vi "Dashboard Main.vi"() -> ()   [LabVIEW 2012]
uses:
  <vilib>/event_ctls.llb/eventvkey.ctl
  <vilib>/Utility/config.llb/Read Key (String).vi
  <vilib>/Utility/config.llb/Read Key (I32).vi
  <vilib>/Utility/config.llb/Write Key (String).vi
  <vilib>/Utility/config.llb/Write Key (I32).vi
  <vilib>/Utility/config.llb/NI_LVConfig.lvlib
panel:
  out "Battery Value":dbl(slide) scale=0.0..14.0 scale format="%#_2e"
  out "Battery":sgl(graph)
  in  "Camera Settings":T1={"Frate Rate"=30, "Compression"=30, "Size"=1} {"Frate Rate" scale=1.0..30.0; "Size" items=["640x480", "320x240", "160x120"]}
  out "Mode":T2(ring)=enum."Auto Disabled"
  out "Camera IP":string
  out "JS1 Z":dbl(slide) scale=-1.0..1.0 scale format="%#_2e"
  out "JS2 Z":dbl(slide) scale=-1.0..1.0 scale format="%#_2e"
  out "Alex Left":cluster{"X":dbl, "Y":dbl}[](graph)
  out "Alex Right":cluster{"X":dbl, "Y":dbl}[](graph)
  out "JS Buttons 1":T3
  out "JS Buttons 2":T3
  out "MotorSlide4":dbl(slide) scale=-1.0..1.0 scale format="%#_2e"
  out "MotorSlide3":dbl(slide) scale=-1.0..1.0 scale format="%#_2e"
  out "MotorSlide2":dbl(slide) scale=-1.0..1.0 scale format="%#_2e"
  in  "MotorName3":string="Front Left"
  in  "MotorName4":string="Front Right"
  in  "MotorName1":string="Rear Left"
  in  "MotorName2":string="Rear Right"
  out "MotorChart4":dbl(graph)
  out "MotorChart3":dbl(graph)
  out "MotorChart2":dbl(graph)
  out "MotorSlide1":dbl(slide) scale=-1.0..1.0 scale format="%#_2e"
  out "MotorChart1":dbl(graph)
  out "Robot IP":string
  in  "Dashboard Tab":enum32{"Operation", "Test", "Checklist"}(tab)
  out "Actual RPM":dbl(knob) max=0.0 scale=-500.0..500.0
  out "At Speed?":bool
  in  "Slider":dbl(slide) scale=0.0..100.0 scale format="%#_3g"
  in  "On/Off":bool caption="Solenoid"
  in  "Test Name":u16(ring) items=["Select the test to run...", "Example Test", "-------------------------------", "List of tests is built in robot code.", "Replace with your own automated tests."]
  in  "Test Tree":string(tree)
  in  "Motor":cluster{"Value":dbl, "Enable":bool} {"Value" scale=-1.0..1.0 scale format="%#_3g"}
  out "Progress":T4 {"Test Progress" scale=0.0..100.0}
  in  "Rev/Fwd":cluster{"Forward":bool, "Reverse":bool}
  in  "Ring":u16(ring) items=["Auto", "Fixed indoor", "Fixed outdoor 1", "Fixed outdoor 2", "Fixed fluorescent 1", "Fixed fluorescent 2", "Hold current"]
  in  "Listbox":i32(listbox)
  in  "Viewer":T5(tab)
  out "Mbps":dbl format="%#.1g"
  in  "Enable":bool
  in  "DB Camera Config":bool
  out "Mbps":bool
  out "fps":dbl format="%#.1g"
  out "Image Error Message":string="Timeout in Camera Communications"
  out "Camera Image":T6(plugin-control)
  out "Buttons 1":cluster{"1":bool, "2":bool, "3":bool}
  out "Kinect 1":cluster{"X":dbl, "Y":dbl, "Z":dbl} {"X" scale=1.0..-1.0; "Y" scale=1.0..-1.0; "Z" scale=1.0..-1.0}
  out "Buttons 2":cluster{"1":bool, "2":bool, "3":bool}
  out "Kinect 2":cluster{"X":dbl, "Y":dbl, "Z":dbl} {"X" scale=1.0..-1.0; "Y" scale=1.0..-1.0; "Z" scale=1.0..-1.0}
  out "Version":string
  out "Skeleton Picture":picture
  out "Players":i8
  out "Tree":string(tree)
  # "Drive & Motors"
  # "Robot IP:"
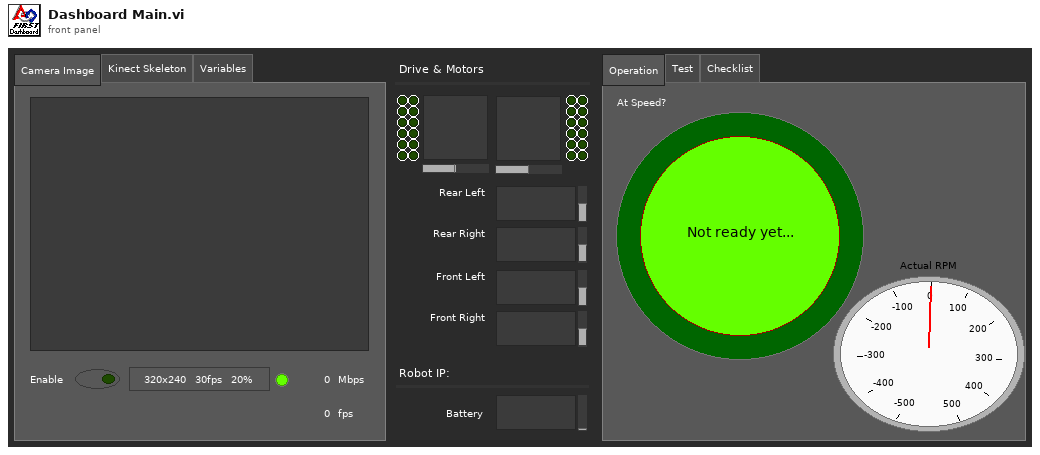
[diagram p1: front panel]
types:
  T1 = cluster{"Frate Rate":i32, "Compression":i32, "Size":u16}
  T2 = enum8{"Tele-Op Disabled", "Tele-Op Enabled", "Auto Disabled", "Auto Enabled", "Test Disabled", "Test Enabled", ""}
  T3 = cluster{bool, bool, bool, bool, bool, bool, bool, bool, bool, bool, bool, bool}
  T4 = cluster{"Test Progress":u8, "Test Progress Text":string}
  T5 = enum32{"Camera Image", "Kinect Skeleton", "Variables"}
  T6 = typedef "IMAQ Image.ctl" = refnum<image>
  T7 = typedef "Image Type" = u32
  T8 = typedef "LVBoundsTypeDef.ctl" = cluster{"Width":u32, "Height":u32}
  T9 = typedef "SkeletonTrackState.ctl" = enum32{"NotTracked", "PositionOnly", "Tracked"}
  T10 = cluster{"TrackingState":u8[], "Position":cluster{"x":sgl, "y":sgl, "z":sgl}, cluster{"x":sgl, "y":sgl, "z":sgl, sgl}[], "TrackState":T9}
  T11 = cluster{cluster{"ScaledToPercentRange":dbl, "ScaledToPercentRange":dbl, "ScaledToPercentRange":dbl}, cluster{bool, bool, bool}}[]
  T12 = cluster{cluster{"ScaledToPercentRange":dbl, "ScaledToPercentRange":dbl, "ScaledToPercentRange":dbl}, cluster{bool, bool, bool}}
  T13 = cluster{"ScaledToPercentRange":dbl, "ScaledToPercentRange":dbl, "ScaledToPercentRange":dbl}
  T14 = typedef "LVRectTypeDef.ctl" = cluster{"Left":i16, "Top":i16, "Right":i16, "Bottom":i16}
  T15 = typedef "NI_LVConfig.lvlib/Config Data RefNum.ctl" = refnum<k1>
  T16 = cluster{"Competition mode":bool, "Robot Link":bool, "Autonomous":bool, "Enabled":bool, "E-Stop":bool, "Simulated":bool, "TestMode":bool, "Docked Window":bool}
  T17 = cluster{"Boolean Array[0]":bool, "Boolean Array[1]":bool, "Boolean Array[2]":bool, "Boolean Array[3]":bool, "Boolean Array[4]":bool, "Boolean Array[5]":bool, "Boolean Array[6]":bool, "Boolean Array[7]":bool, "Boolean Array[8]":bool, "Boolean Array[9]":bool, "Boolean Array[10]":bool, "Boolean Array[11]":bool}
  T18 = typedef "eventvkey.ctl" = enum16{"ASCII", "Enter", "Return", "Shift", "Ctrl", "Alt", "Cmd", "Opt", "Caps", "NumLock", "Clear", "Break", "Up", "Down", "Left", "Right", "Insert", "Delete", "Home", "End", "PageUp", "PageDown", "Escape", "Help", "Pause", "ScrollLock", "F1", "F2", "F3", "F4", "F5", "F6", "F7", "F8", "F9", "F10", "F11", "F12", "F13", "F14", "F15", "F16", "F17", "F18", "F19", "F20", "F21", "F22", "F23", "F24", "Play", "VolumeUp", "VolumeDown", "Mute", "Two Byte Char"}
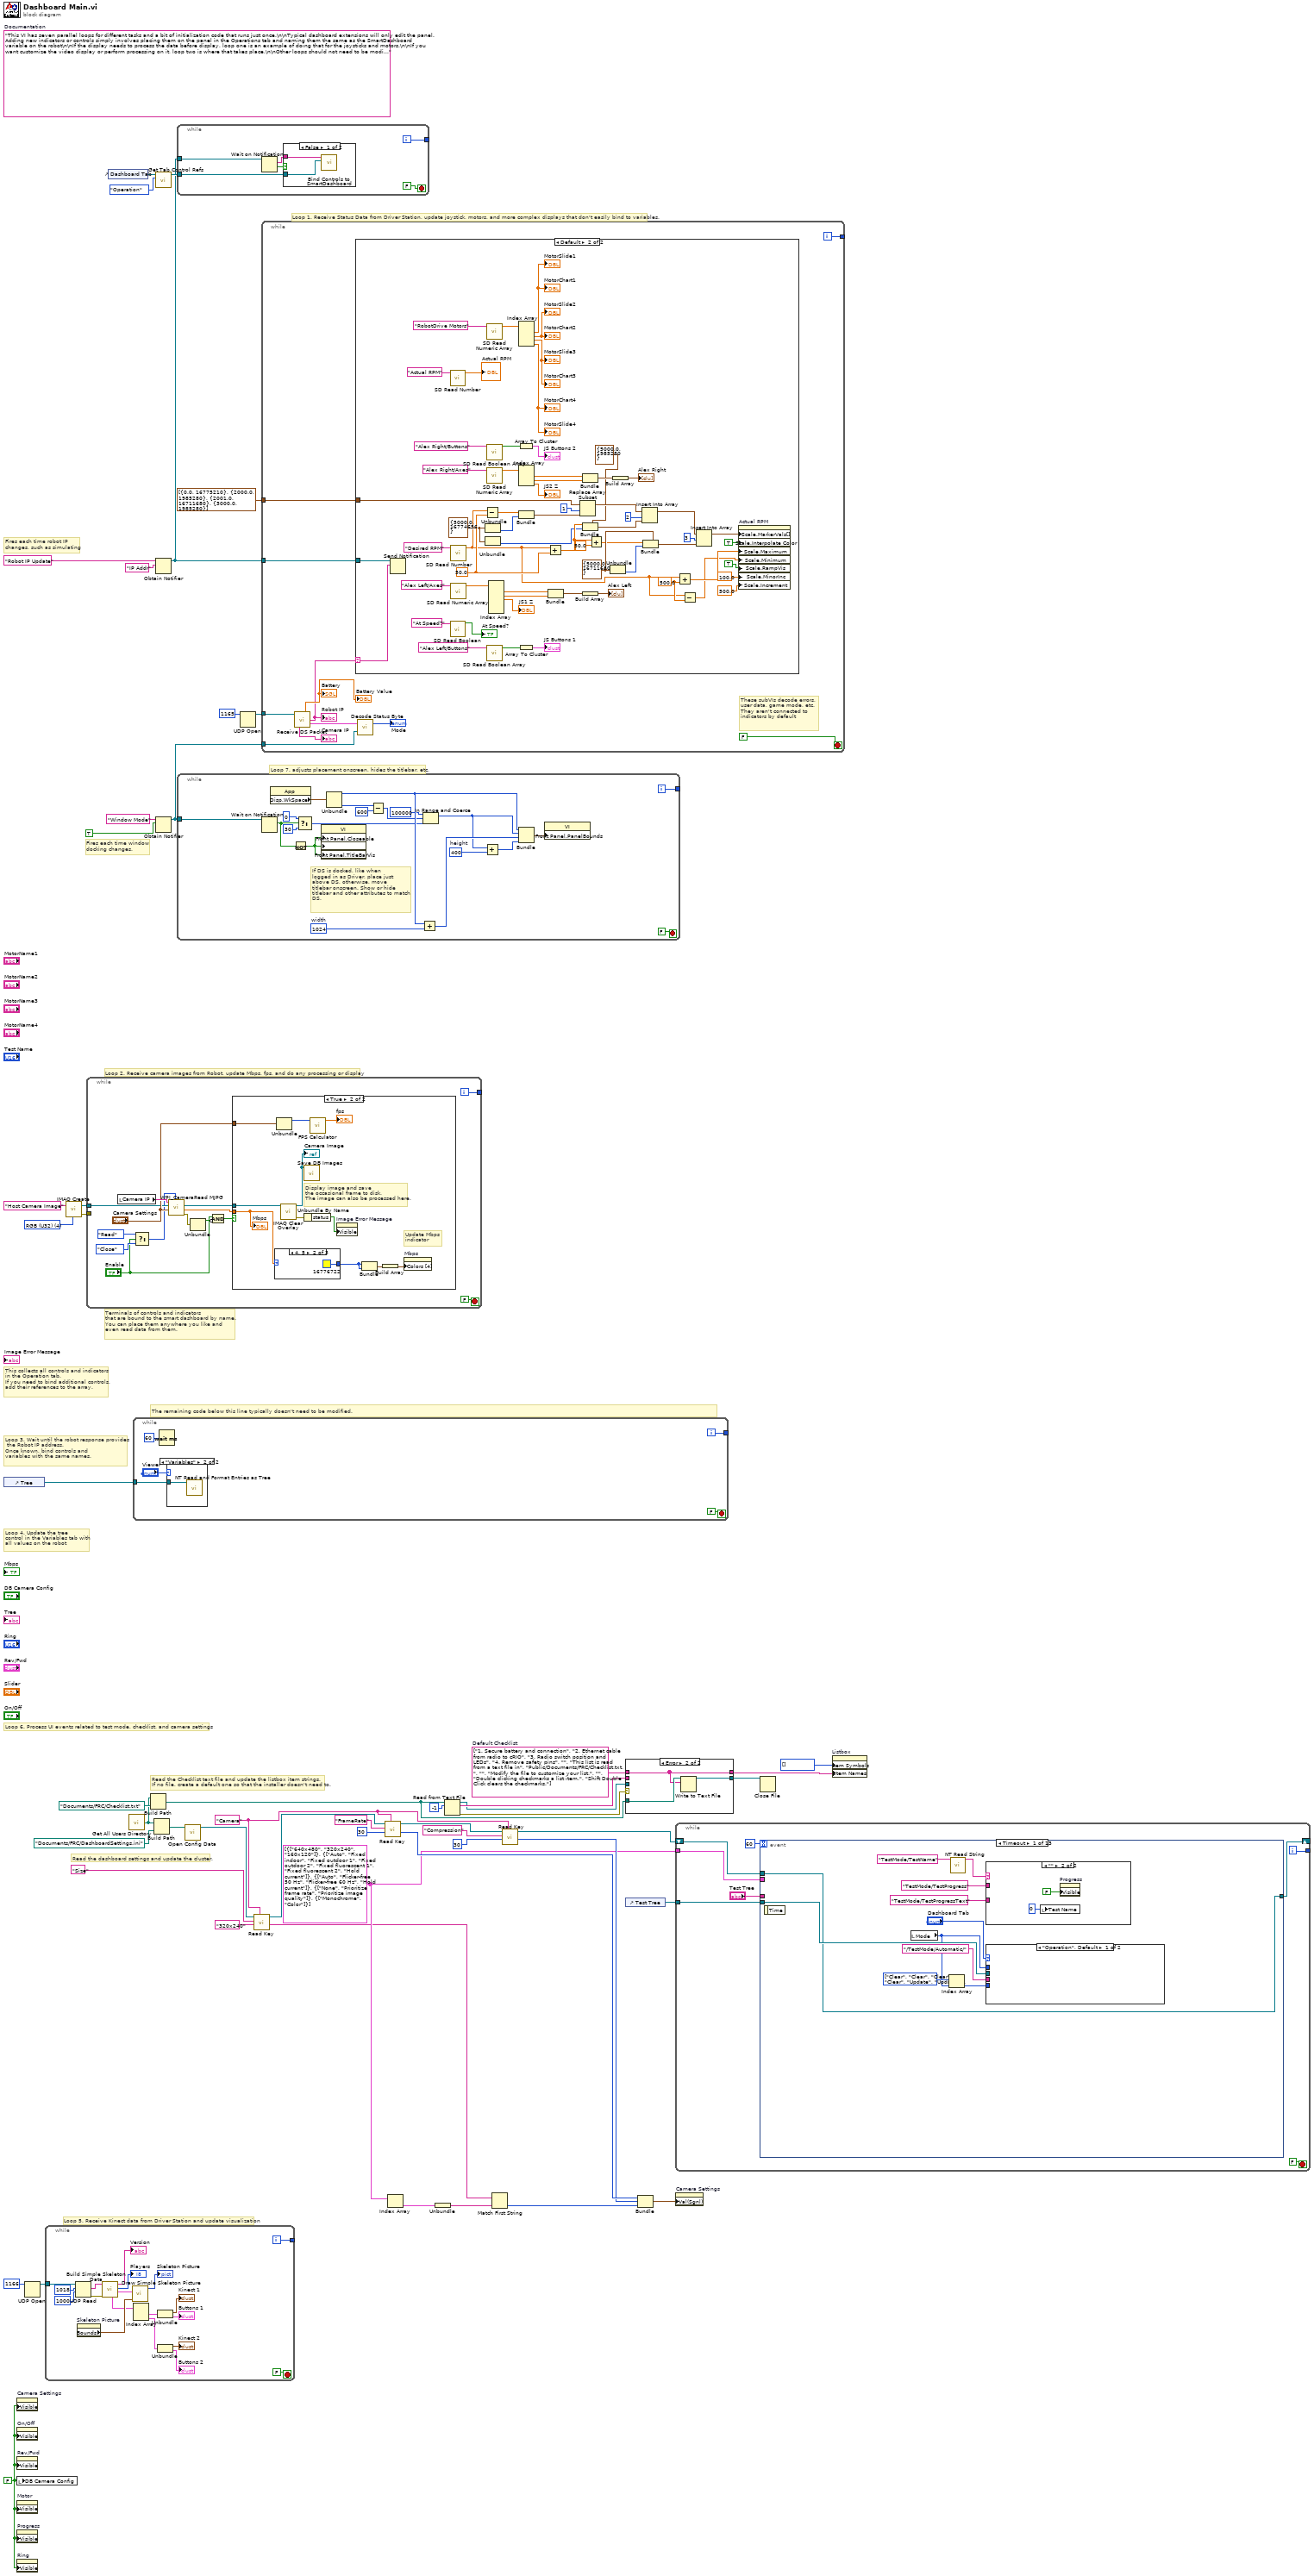
[diagram p0: block diagram]
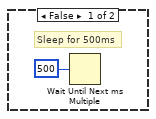
[diagram p3: hidden frame]
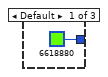
[diagram p4: hidden frame]
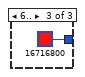
[diagram p5: hidden frame]
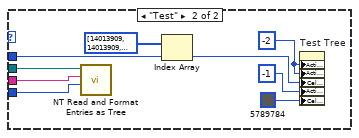
[diagram p7: hidden frame]
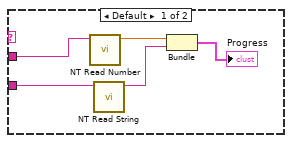
[diagram p8: hidden frame]
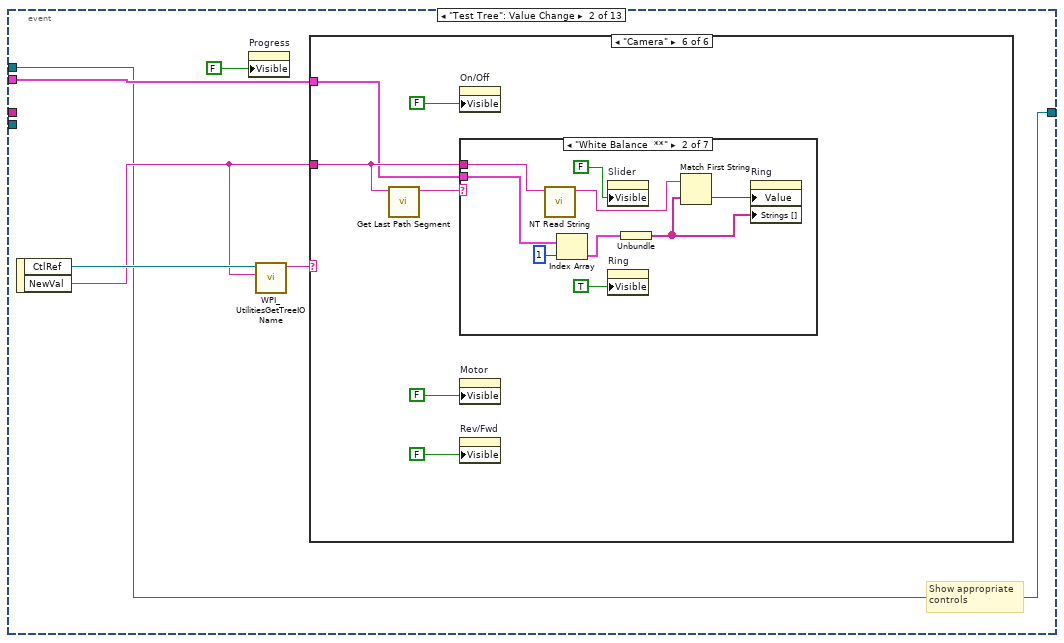
[diagram p9: hidden frame]
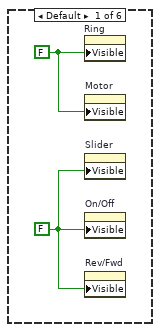
[diagram p10: hidden frame]
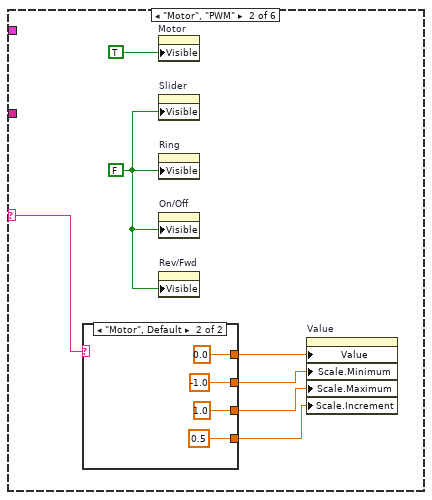
[diagram p11: hidden frame]
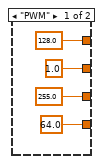
[diagram p12: hidden frame]
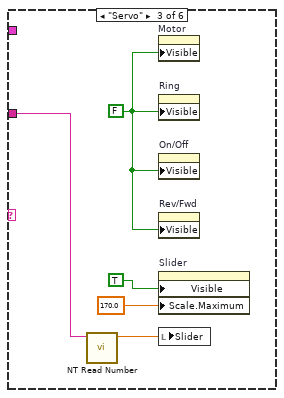
[diagram p13: hidden frame]
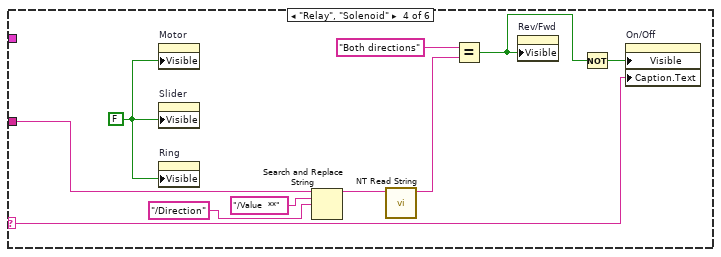
[diagram p14: hidden frame]
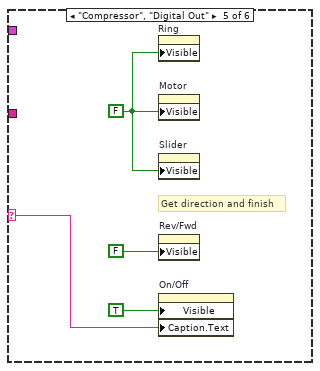
[diagram p15: hidden frame]
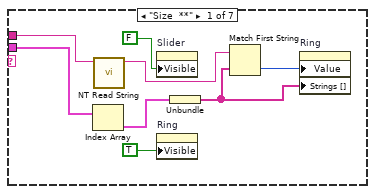
[diagram p16: hidden frame]
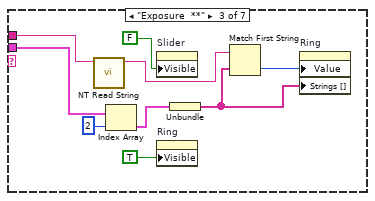
[diagram p17: hidden frame]
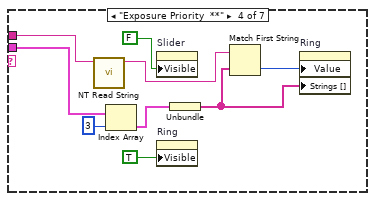
[diagram p18: hidden frame]
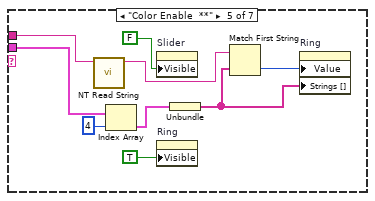
[diagram p19: hidden frame]
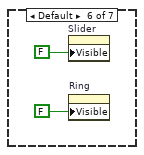
[diagram p20: hidden frame]
diagram:
  w22 = "Camera"
  w14 = cluster{string[]}[] [{["640x480", "320x240", "160x120"]}, {["Auto", "Fixed indoor", "Fixed outdoor 1", "Fixed outdoor 2", "Fixed fluorescent 1", "Fixed fluorescent 2", "Hold current"]}, {["Auto", "Flicker-free 50 Hz", "Flicker-free 60 Hz", "Hold current"]}, {["None", "Prioritize frame rate", "Prioritize image quality"]}, {["Monochrome", "Color"]}]
  w30 = string[] ["1. Secure battery and connection", "2. Ethernet cable from radio to cRIO", "3. Radio switch position and LEDs", "4. Remove safety pins", "", "This list is read from a text file in", "Public/Documents/FRC/Checklist.txt.", "", "Modify the file to customize your list.", "", "Double clicking checkmarks a list item.", "Shift Double Click clears the checkmarks."]  # Default Checklist
  w28 = FALSE ("Visible")
  (unwired) "This VI has seven parallel loops for different tasks and a bit of initialization code that runs just once.\n\nTypical dashboard extensions will only edit the panel. Adding new indicators or controls simply involves placing them on the panel in the Operations tab and naming them the same as the SmartDashboard variable on the robot\n\nIf the display needs to process the data before display, loop one is an example of doing that for the joysticks and motors.\n\nIf you want customize the video display or perform processing on it, loop two is where that takes place.\n\nOther loops should not need to be modified. They are pretty standard, and document the task they perform."  # Documentation
  w51 = T7 4 items=["Grayscale (U8)", "Grayscale (I16)", "Grayscale (SGL)", "Complex (CSG)", "RGB (U32)", "HSL (U32)", "RGB (U64)"] ("Image Type")
  # "Fires each time robot IP\nchanges, such as simulating"
  # "Fires each time window\ndocking changes."
  # "Read the Checklist text file and update the listbox item strings.\nIf no file, create a default one so that the installer doesn't need to."
  # "This collects all controls and indicators\nin the Operation tab.\nIf you need to bind additional controls,\nadd their references to the array."
  # "The remaining code below this line typically doesn't need to be modified."
  # "Loop 6. Process UI events related to test mode, checklist, and camera settings"
  # "Read the dashboard settings and update the cluster."
  # "Terminals of controls and indicators\nthat are bound to the smart dashboard by name.\nYou can place them anywhere you like and\neven read data from them."
  # "Loop 4. Update the tree\ncontrol in the Variables tab with\nall values on the robot"
  # "Loop 3. Wait until the robot response provides\n the Robot IP address.\nOnce known, bind controls and\nvariables with the same names."
  # "Loop 5. Receive Kinect data from Driver Station and update visualization"
  # "Loop 7. adjusts placement onscreen, hides the titlebar, etc."
  # "Loop 1. Receive Status Data from Driver Station, update joystick, motors, and more complex displays that don't easily bind to variables."
  # "Loop 2. Receive camera images from Robot, update Mbps, fps, and do any processing or display"
  n1 = control-ref of="Tree"() -> (w3:refnum<vi>)
  n2 = property on="Camera Settings" class="Clust (strict)"("Visible"=w28) -> ()  [unwired: 2 in, 2 out]
  n3 = property on="On/Off" class="Bool (strict)"("Visible"=w28) -> ()  [unwired: 2 in, 2 out]
  n4 = property on="Rev/Fwd" class="Clust (strict)"("Visible"=w28) -> ()  [unwired: 2 in, 2 out]
  n5 = local write "DB Camera Config"(w28) -> ()
  n6 = property on="Motor" class="Clust (strict)"("Visible"=w28) -> ()  [unwired: 2 in, 2 out]
  n7 = property on="Progress" class="Clust (strict)"("Visible"=w28) -> ()  [unwired: 2 in, 2 out]
  n8 = property on="Ring" class="Ring (strict)"("Visible"=w28) -> ()  [unwired: 2 in, 2 out]
  n9 = UDP Open(11:u16 1166 ("port")) -> (port=w46:refnum<k16>)  [unwired: 2 in, 4 out]
  n10 = while {
    tunnel: w46 -> [w70]
    tunnel: [w55] -> _
    i -> [w55]
    stop <- FALSE stop-if-true
    n11 = UDP Read(connection ID=w70, max size (548)=1018 ("bytes to read"), timeout ms (25000)=1000) -> (data out=w64:string, error out=w54:errorcluster)  [unwired: 1 in, 3 out]
    n12 = property on="Skeleton Picture" class="Pict"() -> ("Bounds"=w66:T8)  [unwired: 2 in, 2 out]
    n13 = call "Build Simple Skeleton Data.vi"("error in (no error)"=w54, "data in"=w64) -> ("Skeleton Data"=w65:T10, "NumPlayers"=→"Players":i8, "Version String"=→"Version":string, "Simple Joystick Info"=w62:T11)  [unwired: 5 in, 1 out]
    n14 = call "Draw Simple Skeleton Picture.vi"("Bounds"=w66, "Simple Skeleton"=w65) -> ("new picture out"=→"Skeleton Picture":picture)  [unwired: 9 in]
    n15 = Index Array(array=w62) -> (element #1=w61:T12, element #2=w60:T12)  [unwired: 2 in]
    n16 = Unbundle(w61) -> (→"Kinect 1":T13, →"Buttons 1":cluster{bool, bool, bool})
    n17 = Unbundle(w60) -> (→"Kinect 2":T13, →"Buttons 2":cluster{bool, bool, bool})
  }
  n18 = call "IMAQ Create"("Image Name"="Host Camera Image", "Image Type"=w51) -> ("New Image"=w49:T6, "error out"=w48:errorcluster)  [unwired: 2 in, 1 out]
  n19 = while {
    tunnel: w49 -> [w82]
    tunnel: w48 -> [_]
    tunnel: [w85] -> _
    i -> [w85]
    stop <- FALSE stop-if-true
    n20 = local read "Camera IP"() -> (w84:string)
    n21 = Select(t=enum16{"Read", "Reopen", "Close"}."Read" ("Operation"), s="Enable", f=enum16{"Read", "Reopen", "Close"}."Close" ("Operation")) -> (s? t:f=w77:enum16{"Read", "Reopen", "Close"})
    n22 = call <vilib>:"WPI_CameraRead MJPG.vi"("Operation"=w77, "Camera Settings"="Camera Settings", "Image"=w82, "address"=w84) -> ("error out"=w76:errorcluster, "Bandwidth (kbps)"=w80:dbl, "Image Out"=w81:T6)  [unwired: 5 in]
    n23 = Unbundle(w76) -> ("status"=w74:bool)  [unwired: 2 out]
    n24 = Compound Arithmetic op=AND("Enable", invert w74) -> (w73:bool)
    n25 = case shown="True" w73 {
      tunnel: "Camera Settings" -> [_ w89]
      tunnel: w81 -> [_ w92]
      tunnel: w80 -> [_ w91]
      frame False {
        # "Sleep for 500ms"
        n26 = Wait Until Next ms Multiple(millisecond multiple=u32 500) -> ()  [unwired: 1 out]
      }
      frame True {
        # "Display image and save\nthe occasional frame to disk.\nThe image can also be processed here."
        # "Update Mbps\nindicator"
        n27 = case shown="4, 5" w91 {
          tunnel: [u32 6618880 ("Color Box") u32 16776722 ("Color Box") u32 16716800 ("Color Box")] -> w93
          frame Default {
          }
          frame 4, 5 {
          }
          frame 6.. {
          }
        }
        n28 = Unbundle(w89) -> ("Frate Rate"=w88:i32)  [unwired: 2 out]
        n29 = call "IMAQ Clear Overlay"("Image"=w92) -> ("error out"=w97:errorcluster, "Image Out"=w96:T6)  [unwired: 2 in, 7 out]
        "Camera Image" <- w96
        n30 = call "Save DB Images.vi"("Image"=w96) -> ()  [unwired: 2 in, 1 out]
        n31 = Unbundle By Name(w97) -> ("status"=w98:bool)
        n32 = call "FPS Calculator.vi"("Average Count"=w88) -> ("fps"=→"fps":dbl)  [unwired: 10 in]
        n33 = property on="Image Error Message" class="Str"("Visible"=w98) -> ()  [unwired: 2 in, 2 out]
        n34 = Bundle("Color Box"=w93, "Color Box"=w93) -> (w95:cluster{"Color Box":u32, "Color Box":u32})  [unwired: 1 out]
        n35 = Build Array(w95) -> (w94:cluster{"Color Box":u32, "Color Box":u32}[])
        n36 = property on="Mbps" class="Bool (strict)"("Colors [4]"=w94) -> ()  [unwired: 2 in, 2 out]
        "Mbps" <- w91
      }
    }
  }
  n37 = control-ref of="Dashboard Tab"() -> (w44:refnum<vi>)
  n38 = call "Get All Users Directory.vi"() -> ("All User Path"=w27:path)
  n39 = while {
    tunnel: [w103] -> _
    tunnel: w3 -> [w102]
    i -> [w103]
    stop <- FALSE stop-if-true
    n40 = Wait (ms)(milliseconds to wait=u32 60) -> ()  [unwired: 1 out]
    n41 = case shown="\"Variables\"" "Viewer" {
      tunnel: w102 -> [_ w107]
      frame Default {
      }
      frame "Variables" {
        n42 = call <vilib>:"NT Read and Format Entries as Tree.vi"("Tree Refnum"=w107) -> ()  [unwired: 9 in, 2 out]
      }
    }
  }
  n43 = Build Path(base path=w27, name or relative path=path "Documents/FRC/Checklist.txt") -> (appended path=w31:path)
  n44 = Build Path(base path=w27, name or relative path=path "Documents/FRC/DashboardSettings.ini") -> (appended path=w26:path)
  n45 = call <vilib>:"Get Tab Control Refs.vi"("Page Index"=enum32{"Operation", "Test"}."Operation" ("Dashboard Tab"), "TabControl in"=w44) -> ("ControlsOnPage"=w45:refnum<vi>[])  [unwired: 9 in]
  n46 = Obtain Notifier(name (unnamed)="Robot IP Update", notification data type="IP Addr" ("name (unnamed)")) -> (notifier out=w41:refnum<notifier>)  [unwired: 2 in, 2 out]
  n47 = Obtain Notifier(name (unnamed)="Window Mode", notification data type=TRUE) -> (notifier out=w34:refnum<notifier>)  [unwired: 2 in, 2 out]
  n48 = while {
    tunnel: w45 -> [w113]
    tunnel: w41 -> [w110]
    tunnel: [w108] -> _
    i -> [w108]
    stop <- FALSE stop-if-true
    n49 = Wait on Notification(notifier=w110) -> (notification=w109:string, timed out?=w111:bool)  [unwired: 3 in, 2 out]
    n50 = case shown="False" w111 {
      tunnel: w113 -> [w115 _]
      tunnel: w109 -> [w114 _]
      frame False {
        n51 = call <vilib>:"Bind Controls to SmartDashboard.vi"("Bound Control Refs"=w115, "Server IP Address"=w114) -> ()  [unwired: 10 in]
      }
      frame True {
      }
    }
  }
  n52 = while {
    tunnel: w34 -> [w134]
    tunnel: [w132] -> _
    i -> [w132]
    stop <- FALSE stop-if-true
    w124 = 1024  # width
    w127 = 400  # height
    # "If DS is docked, like when\nlogged in as Driver, place just\nabove DS, otherwise, move\ntitlebar onscreen. Show or hide\ntitlebar and other attributes to match\nDS."
    n53 = Wait on Notification(notifier=w134) -> (notification=w119:bool)  [unwired: 3 in, 3 out]
    n54 = property class="App"() -> ("Disp.WkSpace"=w130:T14)  [unwired: 2 in, 2 out]
    n55 = Not(x=w119) -> (.not. x?=w133:bool)
    n56 = Select(t=0, s=w119, f=30) -> (s? t:f=w118:i32)
    n57 = property class="VI"("Front Panel.Closeable"=w133, "Front Panel.Minimizeable"=w133, "Front Panel.TitleBarVis"=w133) -> ()  [unwired: 2 in, 2 out]
    n58 = Unbundle(w130) -> ("Left"=w128:i16, "Bottom"=w125:i16)  [unwired: 2 out]
    n59 = Subtract(x=w125, y=600) -> (x-y=w122:i32)
    n60 = Add(x=w128, y=w124) -> (x+y=w129:i32)
    n61 = In Range and Coerce(upper limit=100000, x=w122, lower limit=w118) -> (coerced(x)=w116:i32)  [unwired: 1 out]
    n62 = Add(x=w116, y=w127) -> (x+y=w126:i32)
    n63 = Bundle("Left"=w128, w116, w129, w126) -> (w131:cluster{"Left":i16, i32, i32, i32})  [unwired: 1 out]
    n64 = property class="VI"("Front Panel.PanelBounds"=w131) -> ()  [unwired: 2 in, 2 out]
  }
  n65 = call <vilib>:"Open Config Data.vi"("configuration file path"=w26) -> ("refnum"=w25:T15)  [unwired: 8 in, 2 out]
  n66 = UDP Open(11:u16 1165 ("port")) -> (port=w52:refnum<k16>)  [unwired: 2 in, 4 out]
  n67 = call-poly <vilib>:"Read Key.vi"("section"=w22, "default value"="320x240", "key"="Size", "refnum"=w25) -> ("value"=w12:string, "refnum out"=w7:T15)  [unwired: 2 in, 4 out]
  n68 = while {
    tunnel: w52 -> [w144]
    tunnel: w41 -> [w138]
    tunnel: w34 -> [w142]
    tunnel: [w139] -> _
    tunnel: cluster{dbl, u32}[] [{0.0, 16775210}, {2000.0, 1985280}, {2001.0, 16711680}, {3000.0, 1985280}] ("Scale.Marker Values[]") -> [w136]
    i -> [w139]
    stop <- FALSE stop-if-true
    # "These subVIs decode errors, user data, game mode, etc.\nThey aren't connected to indicators by default"
    n69 = call "Receive DS Packet.vi"("Recv Socket"=w144) -> ("Battery"=→"Battery" →"Battery Value":sgl, "Robot IP Address"=w137:string, "Status"=w145:T16, "Camera IP Address"=→"Camera IP":string)  [unwired: 1 in, 10 out]
    "Robot IP" <- w137
    n70 = case shown="Default" w137 {
      selector: w137 -> [_ w181]
      tunnel: w138 -> [_ w182]
      tunnel: w136 -> [_ w155]
      frame "0.0.0.0" {
        # "Robot not responding, don't poll the variables"
      }
      frame Default {
        w149 = 500.0 ("y")
        w173 = cluster{dbl, u32} {5000.0, 16711680}
        w154 = cluster{dbl, u32} {5000.0, 16774656}
        w162 = 50.0 ("y")
        n71 = Send Notification(notification=w181, notifier=w182) -> ()  [unwired: 1 in, 2 out]
        n72 = call <vilib>:"SD Read Number.vi"("Name"="Actual RPM") -> ("Numeric"=→"Actual RPM":dbl)  [unwired: 8 in, 2 out]
        n73 = call <vilib>:"SD Read Boolean.vi"("Name"="At Speed?") -> ("Boolean"=→"At Speed?":bool)  [unwired: 8 in, 2 out]
        n74 = call <vilib>:"SD Read Number.vi"("Name"="Desired RPM") -> ("Numeric"=w148:dbl)  [unwired: 8 in, 2 out]
        n75 = call <vilib>:"SD Read Numeric Array.vi"("Name"="Alex Left/Axes") -> ("Numeric Array"=w198:dbl[])  [unwired: 8 in, 2 out]
        n76 = Subtract(x=w148, y=w162) -> (x-y=w161:dbl)
        n77 = Unbundle(w154) -> (w159:u32)  [unwired: 1 out]
        n78 = Unbundle(w154) -> (w163:u32)  [unwired: 1 out]
        n79 = call <vilib>:"SD Read Numeric Array.vi"("Name"="RobotDrive Motors") -> ("Numeric Array"=w205:dbl[])  [unwired: 8 in, 2 out]
        n80 = call <vilib>:"SD Read Boolean Array.vi"("Name"="Alex Right/Buttons") -> ("Boolean Array"=w191:bool[])  [unwired: 8 in, 2 out]
        n81 = call <vilib>:"SD Read Numeric Array.vi"("Name"="Alex Right/Axes") -> ("Numeric Array"=w192:dbl[])  [unwired: 8 in, 2 out]
        n82 = call <vilib>:"SD Read Boolean Array.vi"("Name"="Alex Left/Buttons") -> ("Boolean Array"=w200:bool[])  [unwired: 8 in, 2 out]
        n83 = Index Array(array=w198) -> (element #1=w195:dbl, element #2=w196:dbl, element #3=→"JS1 Z":dbl)  [unwired: 6 in, 3 out]
        n84 = Array To Cluster(array=w191) -> (cluster=→"JS Buttons 2":T17)
        n85 = Array To Cluster(array=w200) -> (cluster=→"JS Buttons 1":T17)
        n86 = Index Array(array=w205) -> (element #1=→"MotorChart1" →"MotorSlide1":dbl, element #2=→"MotorSlide2" →"MotorChart2":dbl, element #3=→"MotorChart3" →"MotorSlide3":dbl, element #4=→"MotorChart4" →"MotorSlide4":dbl)  [unwired: 4 in]
        n87 = Index Array(array=w192) -> (element #1=w187:dbl, element #2=w186:dbl, element #3=→"JS2 Z":dbl)  [unwired: 3 in]
        n88 = Bundle(w161, w159) -> (w160:cluster{dbl, u32})  [unwired: 1 in]
        n89 = Add(x=w148, y=w162) -> (x+y=w170:dbl)
        n90 = Bundle("Numeric"=w195, "Numeric"=w196) -> (w194:cluster{"Numeric":dbl, "Numeric":dbl})  [unwired: 1 in]
        n91 = Replace Array Subset(array=w155, new element=w160, index=1) -> (w153:cluster{dbl, u32}[])
        n92 = Bundle("Numeric"=w187, "Numeric"=w186) -> (w188:cluster{"Numeric":dbl, "Numeric":dbl})  [unwired: 1 in]
        n93 = Bundle(cluster=cluster{dbl, u32} {5000.0, 1985280}, w170, w163) -> (w164:cluster{dbl, u32})
        n94 = Build Array(w194) -> (→"Alex Left":cluster{"Numeric":dbl, "Numeric":dbl}[])
        n95 = Add(x=w170, y=50.0) -> (x+y=w172:dbl)
        n96 = Unbundle(w173) -> (w169:u32)  [unwired: 1 out]
        n97 = Build Array(w188) -> (→"Alex Right":cluster{"Numeric":dbl, "Numeric":dbl}[])
        n98 = Insert Into Array(array=w153, index=2, new element=w164) -> (w167:cluster{dbl, u32}[])
        n99 = Bundle(cluster=w173, w172, w169) -> (w174:cluster{dbl, u32})
        n100 = Add(x=w148, y=w149) -> (x+y=w150:dbl)
        n101 = Subtract(x=w148, y=w149) -> (x-y=w147:dbl)
        n102 = Insert Into Array(array=w167, index=3, new element=w174) -> (w152:cluster{dbl, u32}[])
        n103 = property on="Actual RPM" class="Knob (strict)"("Scale.MarkerVals[]"=w152, "Scale.Interpolate Color"=TRUE, "Scale.Maximum"=w150, "Scale.Minimum"=w147, "Scale.RampVis"=TRUE ("Scale.Ramp Visible"), "Scale.MinorInc"=100.0 ("Scale.Range:Minor Increment"), "Scale.Increment"=500.0 ("Scale.Range:Increment")) -> ()  [unwired: 2 in, 2 out]
      }
    }
    n104 = call "Decode Status Byte.vi"("Window Mode Notifier"=w142, "Status"=w145) -> ("Mode"=→"Mode":T2)  [unwired: 1 out]
  }
  n105 = call-poly <vilib>:"Read Key.vi"("section"=w22, "default value"=30, "key"="FrameRate", "refnum"=w7) -> ("value"=w17:i32, "refnum out"=w6:T15)  [unwired: 1 in, 5 out]
  n106 = Index Array(array=w14) -> (element=w15:cluster{string[]})  [unwired: 1 in]
  n107 = Unbundle(w15) -> (w13:string[])
  n108 = Read from Text File(file (use dialog)=w31, count=-1 ("timeout ms (25000)")) -> (refnum out=w9:refnum<file>, text=w32:string[], error out=w33:errorcluster)  [unwired: 2 in, 1 out]
  n109 = Match First String(2:w13, 3:w12) -> (0:w11:i32)  [unwired: 1 out]
  n110 = call-poly <vilib>:"Read Key.vi"("section"=w22, "default value"=30, "key"="Compression", "refnum"=w6) -> ("value"=w16:i32, "refnum out"=w4:T15)  [unwired: 1 in, 5 out]
  n111 = case shown="Error" w33 {
    tunnel: w32 -> [w210 _]
    tunnel: [w210 w212] -> w29
    tunnel: w30 -> [_ w212]
    tunnel: w31 -> [_ w213]
    tunnel: [w209 w211] -> w8
    tunnel: w9 -> [w209 _]
    frame No Error {
    }
    frame Error {
      n112 = Write to Text File(file (use dialog)=w213, text=w212) -> (refnum out=w211:refnum<file>)  [unwired: 2 in, 2 out]
    }
  }
  n113 = control-ref of="Test Tree"() -> (w2:refnum<vi>)
  n114 = Bundle("value"=w17, "value"=w16, "index"=w11) -> (w5:cluster{"value":i32, "value":i32, "index":i32})  [unwired: 1 out]
  n115 = while {
    tunnel: w14 -> [w218]
    shift-right: [w217] -> _
    shift-left: w4 -> [w216]
    tunnel: [w215] -> _
    tunnel: w2 -> [w214]
    i -> [w215]
    stop <- FALSE stop-if-true
    n116 = event shown="[0] Timeout" {
      selector: _ -> [_ _ _ _ _ _ _ _ _ _ _ _ _]
      dyn-events: _ -> [_ _ _ _ _ _ _ _ _ _ _ _ _]
      timeout: u32 60 ("milliseconds to wait") -> [_ _ _ _ _ _ _ _ _ _ _ _ _]
      tunnel: w214 -> [w228 _ _ _ _ _ _ _ _ _ _ _ _]
      tunnel: "Test Tree" -> [_ _ _ _ _ _ _ _ w422 w430 w432 w436 w444]
      tunnel: w218 -> [_ w250 _ _ _ _ w386 w416 _ _ _ _ _]
      tunnel: [w222 w249 _ w352 w360 w372 w385 w409 w421 w428 w431 w435 w443] -> w217
      tunnel: w216 -> [w222 w249 _ w352 w360 w372 w384 w409 w421 w428 w431 w435 w443]
      event Timeout {
        w227 = enum16{"Update", "Clear"}[] [enum."Clear", enum."Clear", enum."Clear", enum."Clear", enum."Update", enum."Update", enum."Clear"] items=["Update", "Clear"]
        n117 = event-data() -> ()  [unwired: 1 in, 1 out]
        n118 = local read "Mode"() -> (w225:T2)
        n119 = Index Array(array=w227, index=w225) -> (element=w226:enum16{"Update", "Clear"})
        n120 = call <vilib>:"NT Read String.vi"("Name"="TestMode/TestName") -> ("String"=w231:string)  [unwired: 9 in, 1 out]
        n121 = case shown="\"\"" w231 {
          tunnel: "TestMode/TestProgress" ("Name") -> [w243 _]
          tunnel: "TestMode/TestProgressText" ("Name") -> [w242 _]
          frame Default {
            n122 = call <vilib>:"NT Read Number.vi"("Name"=w243) -> ("Numeric"=w244:dbl)  [unwired: 9 in, 1 out]
            n123 = call <vilib>:"NT Read String.vi"("Name"=w242) -> ("String"=w245:string)  [unwired: 9 in, 1 out]
            n124 = Bundle("Numeric"=w244, "String"=w245) -> (→"Progress":cluster{"Numeric":dbl, "String":string})  [unwired: 1 in]
          }
          frame "" {
            n125 = local write "Test Name"(u16 0) -> ()
            n126 = property on="Progress" class="Clust (strict)"("Visible"=FALSE) -> ()  [unwired: 2 in, 2 out]
          }
        }
        n127 = case shown="\"Operation\", Default" "Dashboard Tab" {
          tunnel: w228 -> [_ w241]
          tunnel: "/TestMode/Automatic/" ("Name Pattern") -> [_ w240]
          tunnel: w226 -> [_ w239]
          tunnel: w225 -> [_ w237]
          frame "Operation", Default {
          }
          frame "Test" {
            w236 = -2 ("Active Item:Row Number")
            n128 = call <vilib>:"NT Read and Format Entries as Tree.vi"("Operation"=w239, "Name Pattern"=w240, "Tree Refnum"=w241) -> ()  [unwired: 7 in, 2 out]
            n129 = Index Array(array=u32[] [14013909, 14013909, 14013909, 14013909, 14013909, 16777215, 14013909], index=w237) -> (element=w235:u32)
            n130 = property on="Test Tree" class="Tree (strict)"("Active Item Row Number"=w236, "ActiveColNum"=w236, "CellBG"=w235, "Active Item Row Number"=-1 ("Active Item:Row Number"), "CellBG"=u32 5789784 ("Color Box")) -> ()  [unwired: 2 in, 2 out]
          }
        }
      }
      event "Test Tree": Value Change {
        # "Show appropriate\ncontrols"
        n131 = event-data() -> ("CtlRef"=w253:refnum<vi>, "NewVal"=w251:string)  [unwired: 1 in]
        n132 = property on="Progress" class="Clust (strict)"("Visible"=FALSE) -> ()  [unwired: 2 in, 2 out]
        n133 = call <vilib>:"WPI_UtilitiesGetTreeIOName.vi"("NewVal"=w251, "TreeControl in"=w253) -> ("I/O Name"=w254:string)  [unwired: 9 in]
        n134 = case shown="\"Camera\"" w254 {
          selector: w254 -> [_ w261 _ w279 w288 _]
          tunnel: w251 -> [_ _ w276 w278 _ w295]
          tunnel: w250 -> [_ _ _ _ _ w294]
          frame Default {
            w256 = FALSE ("Visible")
            w255 = FALSE ("Visible")
            n135 = property on="Ring" class="Ring (strict)"("Visible"=w255) -> ()  [unwired: 2 in, 2 out]
            n136 = property on="Motor" class="Clust (strict)"("Visible"=w255) -> ()  [unwired: 2 in, 2 out]
            n137 = property on="Slider" class="Slide (strict)"("Visible"=w256) -> ()  [unwired: 2 in, 2 out]
            n138 = property on="On/Off" class="Bool (strict)"("Visible"=w256) -> ()  [unwired: 2 in, 2 out]
            n139 = property on="Rev/Fwd" class="Clust (strict)"("Visible"=w256) -> ()  [unwired: 2 in, 2 out]
          }
          frame "Motor", "PWM" {
            w262 = FALSE ("Visible")
            n140 = case shown="\"Motor\", Default" w261 {
              tunnel: [1.0 ("Value") -1.0 ("Value")] -> w260
              tunnel: [255.0 ("Value") 1.0 ("Value")] -> w259
              tunnel: [128.0 ("Value") 0.0 ("Value")] -> w258
              tunnel: [64.0 ("Value") 0.5 ("Value")] -> w257
              frame "PWM" {
              }
              frame "Motor", Default {
              }
            }
            n141 = property on="Motor" class="Clust (strict)"("Visible"=TRUE) -> ()  [unwired: 2 in, 2 out]
            n142 = property on="Slider" class="Slide (strict)"("Visible"=w262) -> ()  [unwired: 2 in, 2 out]
            n143 = property on="Ring" class="Ring (strict)"("Visible"=w262) -> ()  [unwired: 2 in, 2 out]
            n144 = property on="On/Off" class="Bool (strict)"("Visible"=w262) -> ()  [unwired: 2 in, 2 out]
            n145 = property on="Rev/Fwd" class="Clust (strict)"("Visible"=w262) -> ()  [unwired: 2 in, 2 out]
            n146 = property on="Value" class="Slide (strict)"("Value"=w258, "Scale.Minimum"=w260, "Scale.Maximum"=w259, "Scale.Increment"=w257) -> ()  [unwired: 2 in, 2 out]
          }
          frame "Servo" {
            w274 = FALSE ("Visible")
            n147 = call <vilib>:"NT Read Number.vi"("Name"=w276) -> ("Numeric"=w275:dbl)  [unwired: 9 in, 1 out]
            n148 = property on="Motor" class="Clust (strict)"("Visible"=w274) -> ()  [unwired: 2 in, 2 out]
            n149 = property on="Ring" class="Ring (strict)"("Visible"=w274) -> ()  [unwired: 2 in, 2 out]
            n150 = property on="On/Off" class="Bool (strict)"("Visible"=w274) -> ()  [unwired: 2 in, 2 out]
            n151 = property on="Rev/Fwd" class="Clust (strict)"("Visible"=w274) -> ()  [unwired: 2 in, 2 out]
            n152 = property on="Slider" class="Slide (strict)"("Visible"=TRUE, "Scale.Maximum"=170.0 ("Scale.Range:Maximum")) -> ()  [unwired: 2 in, 2 out]
            n153 = local write "Slider"(w275) -> ()
          }
          frame "Relay", "Solenoid" {
            w277 = FALSE ("Visible")
            n154 = property on="Motor" class="Clust (strict)"("Visible"=w277) -> ()  [unwired: 2 in, 2 out]
            n155 = property on="Slider" class="Slide (strict)"("Visible"=w277) -> ()  [unwired: 2 in, 2 out]
            n156 = property on="Ring" class="Ring (strict)"("Visible"=w277) -> ()  [unwired: 2 in, 2 out]
            n157 = Search and Replace String(input string=w278, search string="/Value  **", replace string="/Direction") -> (result string=w284:string)  [unwired: 5 in, 3 out]
            n158 = call <vilib>:"NT Read String.vi"("Name"=w284) -> ("String"=w282:string)  [unwired: 9 in, 1 out]
            n159 = Equal?(x="Both directions", y=w282) -> (x = y?=w280:bool)
            n160 = property on="Rev/Fwd" class="Clust (strict)"("Visible"=w280) -> ()  [unwired: 2 in, 2 out]
            n161 = Not(x=w280) -> (.not. x?=w281:bool)
            n162 = property on="On/Off" class="Bool (strict)"("Visible"=w281, "Caption.Text"=w279) -> ()  [unwired: 2 in, 2 out]
          }
          frame "Compressor", "Digital Out" {
            w287 = FALSE ("Visible")
            # "Get direction and finish"
            n163 = property on="Ring" class="Ring (strict)"("Visible"=w287) -> ()  [unwired: 2 in, 2 out]
            n164 = property on="Motor" class="Clust (strict)"("Visible"=w287) -> ()  [unwired: 2 in, 2 out]
            n165 = property on="Slider" class="Slide (strict)"("Visible"=w287) -> ()  [unwired: 2 in, 2 out]
            n166 = property on="Rev/Fwd" class="Clust (strict)"("Visible"=FALSE) -> ()  [unwired: 2 in, 2 out]
            n167 = property on="On/Off" class="Bool (strict)"("Visible"=TRUE, "Caption.Text"=w288) -> ()  [unwired: 2 in, 2 out]
          }
          frame "Camera" {
            n168 = call <vilib>:"Get Last Path Segment.vi"("String in"=w295) -> ("String out"=w296:string)  [unwired: 10 in]
            n169 = property on="On/Off" class="Bool (strict)"("Visible"=FALSE) -> ()  [unwired: 2 in, 2 out]
            n170 = case shown="\"White Balance  **\"" w296 {
              tunnel: w295 -> [w302 w311 w320 w329 w338 _ w344]
              tunnel: w294 -> [w300 w308 w317 w326 w335 _ _]
              frame "Size  **" {
                n171 = Index Array(array=w300) -> (element=w299:cluster{string[]})  [unwired: 1 in]
                n172 = call <vilib>:"NT Read String.vi"("Name"=w302) -> ("String"=w301:string)  [unwired: 9 in, 1 out]
                n173 = property on="Slider" class="Slide (strict)"("Visible"=FALSE) -> ()  [unwired: 2 in, 2 out]
                n174 = property on="Ring" class="Ring (strict)"("Visible"=TRUE) -> ()  [unwired: 2 in, 2 out]
                n175 = Unbundle(w299) -> (w297:string[])
                n176 = Match First String(2:w297, 3:w301) -> (0:w298:i32)  [unwired: 1 out]
                n177 = property on="Ring" class="Ring (strict)"("Value"=w298, "Strings []"=w297) -> ()  [unwired: 2 in, 2 out]
              }
              frame "White Balance  **" {
                n178 = call <vilib>:"NT Read String.vi"("Name"=w311) -> ("String"=w310:string)  [unwired: 9 in, 1 out]
                n179 = Index Array(array=w308, index=1) -> (element=w309:cluster{string[]})
                n180 = property on="Slider" class="Slide (strict)"("Visible"=FALSE) -> ()  [unwired: 2 in, 2 out]
                n181 = property on="Ring" class="Ring (strict)"("Visible"=TRUE) -> ()  [unwired: 2 in, 2 out]
                n182 = Unbundle(w309) -> (w306:string[])
                n183 = Match First String(2:w306, 3:w310) -> (0:w305:i32)  [unwired: 1 out]
                n184 = property on="Ring" class="Ring (strict)"("Value"=w305, "Strings []"=w306) -> ()  [unwired: 2 in, 2 out]
              }
              frame "Exposure  **" {
                n185 = call <vilib>:"NT Read String.vi"("Name"=w320) -> ("String"=w319:string)  [unwired: 9 in, 1 out]
                n186 = Index Array(array=w317, index=2) -> (element=w318:cluster{string[]})
                n187 = property on="Slider" class="Slide (strict)"("Visible"=FALSE) -> ()  [unwired: 2 in, 2 out]
                n188 = property on="Ring" class="Ring (strict)"("Visible"=TRUE) -> ()  [unwired: 2 in, 2 out]
                n189 = Unbundle(w318) -> (w314:string[])
                n190 = Match First String(2:w314, 3:w319) -> (0:w315:i32)  [unwired: 1 out]
                n191 = property on="Ring" class="Ring (strict)"("Value"=w315, "Strings []"=w314) -> ()  [unwired: 2 in, 2 out]
              }
              frame "Exposure Priority  **" {
                n192 = call <vilib>:"NT Read String.vi"("Name"=w329) -> ("String"=w328:string)  [unwired: 9 in, 1 out]
                n193 = Index Array(array=w326, index=3) -> (element=w327:cluster{string[]})
                n194 = property on="Slider" class="Slide (strict)"("Visible"=FALSE) -> ()  [unwired: 2 in, 2 out]
                n195 = property on="Ring" class="Ring (strict)"("Visible"=TRUE) -> ()  [unwired: 2 in, 2 out]
                n196 = Unbundle(w327) -> (w323:string[])
                n197 = Match First String(2:w323, 3:w328) -> (0:w324:i32)  [unwired: 1 out]
                n198 = property on="Ring" class="Ring (strict)"("Value"=w324, "Strings []"=w323) -> ()  [unwired: 2 in, 2 out]
              }
              frame "Color Enable  **" {
                n199 = call <vilib>:"NT Read String.vi"("Name"=w338) -> ("String"=w337:string)  [unwired: 9 in, 1 out]
                n200 = Index Array(array=w335, index=4) -> (element=w336:cluster{string[]})
                n201 = property on="Slider" class="Slide (strict)"("Visible"=FALSE) -> ()  [unwired: 2 in, 2 out]
                n202 = property on="Ring" class="Ring (strict)"("Visible"=TRUE) -> ()  [unwired: 2 in, 2 out]
                n203 = Unbundle(w336) -> (w332:string[])
                n204 = Match First String(2:w332, 3:w337) -> (0:w333:i32)  [unwired: 1 out]
                n205 = property on="Ring" class="Ring (strict)"("Value"=w333, "Strings []"=w332) -> ()  [unwired: 2 in, 2 out]
              }
              frame Default {
                n206 = property on="Slider" class="Slide (strict)"("Visible"=FALSE) -> ()  [unwired: 2 in, 2 out]
                n207 = property on="Ring" class="Ring (strict)"("Visible"=FALSE) -> ()  [unwired: 2 in, 2 out]
              }
              frame "Brightness  **", "Color Level  **", "Compression  **", "FPS  **", "Sharpness  **" {
                n208 = call <vilib>:"NT Read Number.vi"("Name"=w344) -> ("Numeric"=w343:dbl)  [unwired: 9 in, 1 out]
                n209 = property on="Ring" class="Ring (strict)"("Visible"=FALSE) -> ()  [unwired: 2 in, 2 out]
                n210 = property on="Slider" class="Slide (strict)"("Visible"=TRUE, "Scale.Maximum"=100.0 ("Scale.Range:Maximum")) -> ()  [unwired: 2 in, 2 out]
                n211 = local write "Slider"(w343) -> ()
              }
            }
            n212 = property on="Motor" class="Clust (strict)"("Visible"=FALSE) -> ()  [unwired: 2 in, 2 out]
            n213 = property on="Rev/Fwd" class="Clust (strict)"("Visible"=FALSE) -> ()  [unwired: 2 in, 2 out]
          }
        }
      }
      event "Test Name": Mouse Enter {
        # "Populate the ring with the list of tests"
        n214 = event-data() -> ()  [unwired: 1 in, 1 out]
        n215 = call <vilib>:"NT Read String Array.vi"("Name"="TestMode/TestList") -> ("String Array"=w351:string[])  [unwired: 9 in, 1 out]
        n216 = Build Array (concatenate)("Select the test to run...", w351) -> (w350:string[])
        n217 = property on="Test Name" class="Ring (strict)"("Strings []"=w350) -> ()  [unwired: 2 in, 2 out]
      }
      event "Test Name": Value Change {
        w353 = FALSE ("Visible")
        # "Tell the robot the test name to run"
        n218 = event-data() -> ("NewVal"=w357:u16)  [unwired: 1 in]
        n219 = property on="Test Name" class="Ring (strict)"() -> ("Strings []"=w358:string[])  [unwired: 2 in, 2 out]
        n220 = property on="Ring" class="Ring (strict)"("Visible"=w353) -> ()  [unwired: 2 in, 2 out]
        n221 = property on="Motor" class="Clust (strict)"("Visible"=w353) -> ()  [unwired: 2 in, 2 out]
        n222 = property on="Slider" class="Slide (strict)"("Visible"=w353) -> ()  [unwired: 2 in, 2 out]
        n223 = property on="On/Off" class="Bool (strict)"("Visible"=w353) -> ()  [unwired: 2 in, 2 out]
        n224 = property on="Rev/Fwd" class="Clust (strict)"("Visible"=w353) -> ()  [unwired: 2 in, 2 out]
        n225 = local write "Progress"(T4 {"Test Progress"=0, "Test Progress Text"=""} ("Progress")) -> ()
        n226 = property on="Progress" class="Clust (strict)"("Visible"=TRUE) -> ()  [unwired: 2 in, 2 out]
        n227 = Index Array(array=w358, index=w357) -> (element=w356:string)
        n228 = call <vilib>:"NT Write String.vi"("String"=w356, "Name"="TestMode/TestName") -> ()  [unwired: 9 in, 1 out]
      }
      event "Listbox": Double Click {
        n229 = event-data() -> ("PlatMods.Shift"=w361:bool, "Row"=w363:i32)  [unwired: 1 in]
        n230 = case shown="False" w361 {
          tunnel: w363 -> [w367 _]
          tunnel: 1 -> [w366 _]
          frame False {
            n231 = property on="Listbox" class="LstBox (strict)"() -> ("Item Symbols"=w365:i32[])  [unwired: 2 in, 2 out]
            n232 = Replace Array Subset(array=w365, new element=w366, index=w367) -> (w364:i32[])
            n233 = property on="Listbox" class="LstBox (strict)"("Item Symbols"=w364) -> ()  [unwired: 2 in, 2 out]
          }
          frame True {
            w368 = 0 ("Top Row")
            n234 = property on="Listbox" class="LstBox (strict)"() -> ("Number of Rows"=w370:u32)  [unwired: 2 in, 2 out]
            n235 = Initialize Array(0, w370) -> (w369:i32[])
            n236 = property on="Listbox" class="LstBox (strict)"("Top Row"=w368, "Value"=w368, "Item Symbols"=w369) -> ()  [unwired: 2 in, 2 out]
          }
        }
      }
      event "Listbox": Key Down {
        n237 = event-data() -> ("VKey"=w374:T18)  [unwired: 1 in]
        n238 = case shown="\"Left\", \"Right\"" w374 {
          selector: w374 -> [w379 _]
          tunnel: eventvkey."Left" ("VKey") -> [w377 _]
          frame "Left", "Right" {
            n239 = Equal?(x=w377, y=w379) -> (x = y?=w378:bool)
            n240 = Select(t=0, s=w378, f=1) -> (s? t:f=w380:i32)
            n241 = property on="Listbox" class="LstBox (strict)"() -> ("Item Symbols"=w383:i32[])  [unwired: 2 in, 2 out]
            n242 = Replace Array Subset(array=w383, new element=w380, index="Listbox") -> (w382:i32[])
            n243 = property on="Listbox" class="LstBox (strict)"("Item Symbols"=w382) -> ()  [unwired: 2 in, 2 out]
          }
          frame Default {
          }
        }
      }
      event "DB Camera Config": Value Change {
        n244 = event-data() -> ("NewVal"=w387:bool)  [unwired: 1 in]
        n245 = case shown="False" w387 {
          tunnel: w386 -> [w396 _]
          tunnel: [w389 w407] -> w385
          tunnel: w384 -> [w388 w407]
          frame False {
            w403 = "Camera"
            w406 = FALSE ("Visible")
            n246 = property on="Camera Settings" class="Clust (strict)"("Visible"=w406) -> ()  [unwired: 2 in, 2 out]
            n247 = local write "DB Camera Config"(w406) -> ()
            n248 = local read "Camera Settings"() -> (w395:T1)
            n249 = Index Array(array=w396) -> (element=w399:cluster{string[]})  [unwired: 1 in]
            n250 = Unbundle(w399) -> (w398:string[])
            n251 = Unbundle(w395) -> ("Frate Rate"=w394:i32, "Compression"=w393:i32, "Size"=w397:u16)
            n252 = Index Array(array=w398, index=w397) -> (element=w392:string)
            n253 = call-poly <vilib>:"Write Key.vi"("section"=w403, "value"=w392, "key"="Size", "refnum"=w388) -> ("refnum out"=w405:T15)  [unwired: 2 in, 5 out]
            n254 = call-poly <vilib>:"Write Key.vi"("section"=w403, "value"=w394, "key"="FrameRate", "refnum"=w405) -> ("refnum out"=w404:T15)  [unwired: 1 in, 6 out]
            n255 = call-poly <vilib>:"Write Key.vi"("section"=w403, "value"=w393, "key"="Compression", "refnum"=w404) -> ("refnum out"=w390:T15)  [unwired: 1 in, 6 out]
            n256 = call <vilib>:"Close Config Data.vi"("refnum"=w390) -> ("file path"=w391:path)  [unwired: 2 in, 8 out]
            n257 = call <vilib>:"Open Config Data.vi"("configuration file path"=w391) -> ("refnum"=w389:T15)  [unwired: 8 in, 2 out]
          }
          frame True {
            n258 = property on="Camera Settings" class="Clust (strict)"("Visible"=TRUE) -> ()  [unwired: 2 in, 2 out]
          }
        }
      }
      event "Camera Settings": Value Change {
        n259 = event-data() -> ("NewVal"=w420:T1)  [unwired: 1 in]
        n260 = Index Array(array=w416) -> (element=w415:cluster{string[]})  [unwired: 1 in]
        n261 = Unbundle(w415) -> (w414:string[])
        n262 = Unbundle(w420) -> ("Frate Rate"=w411:i32, "Compression"=w410:i32, "Size"=w413:u16)
        n263 = Index Array(array=w414, index=w413) -> (element=w412:string)
        n264 = Format Into String(format string="%s   %dfps   %d%%", w412, w411, w410) -> (resulting string=w417:string)  [unwired: 2 in, 1 out]
        n265 = Build Array(w417) -> (w418:string[])
        n266 = property on="DB Camera Config" class="Bool (strict)"("Strings [4]"=w418) -> ()  [unwired: 2 in, 2 out]
      }
      event "Motor.Enable": Value Change {
        n267 = event-data() -> ("NewVal"=w426:bool)  [unwired: 1 in]
        n268 = Unbundle("Motor") -> ("Value"=w425:dbl)  [unwired: 1 out]
        n269 = Select(t=w425, s=w426, f=0.0) -> (s? t:f=w423:dbl)
        n270 = call <vilib>:"NT Write Number.vi"("Numeric"=w423, "Name"=w422) -> ()  [unwired: 9 in, 1 out]
      }
      event "Slider": Value Change {
        n271 = event-data() -> ("NewVal"=w429:dbl)  [unwired: 1 in]
        n272 = call <vilib>:"NT Write Number.vi"("Numeric"=w429, "Name"=w430) -> ()  [unwired: 9 in, 1 out]
      }
      event "On/Off": Value Change {
        n273 = event-data() -> ("NewVal"=w434:bool)  [unwired: 1 in]
        n274 = Boolean To (0,1)(Boolean=w434) -> (0, 1=w433:i16)
        n275 = call <vilib>:"NT Write Number.vi"("Numeric"=w433, "Name"=w432) -> ()  [unwired: 9 in, 1 out]
      }
      event "Rev/Fwd": Value Change {
        n276 = event-data() -> ("NewVal.Forward"=w442:bool, "NewVal.Reverse"=w441:bool)  [unwired: 1 in]
        n277 = Boolean To (0,1)(Boolean=w441) -> (0, 1=w440:i16)
        n278 = Boolean To (0,1)(Boolean=w442) -> (0, 1=w438:i16)
        n279 = Negate(x=w440) -> (-x=w439:i16)
        n280 = Add(x=w438, y=w439) -> (x+y=w437:i16)
        n281 = call <vilib>:"NT Write Number.vi"("Numeric"=w437, "Name"=w436) -> ()  [unwired: 9 in, 1 out]
      }
      event "Ring": Value Change {
        n282 = event-data() -> ("NewVal"=w446:u16)  [unwired: 1 in]
        n283 = property on="Ring" class="Ring (strict)"() -> ("Strings []"=w447:string[])  [unwired: 2 in, 2 out]
        n284 = Index Array(array=w447, index=w446) -> (element=w445:string)
        n285 = call <vilib>:"NT Write String.vi"("String"=w445, "Name"=w444) -> ()  [unwired: 9 in, 1 out]
      }
    }
  }
  n286 = property on="Camera Settings" class="Clust (strict)"("Val(Sgnl)"=w5) -> ()  [unwired: 2 in, 2 out]
  n287 = Close File(refnum=w8) -> ()  [unwired: 1 in, 2 out]
  n288 = property on="Listbox" class="LstBox (strict)"("Item Symbols"=i32[] [], "Item Names"=w29) -> ()  [unwired: 2 in, 2 out]
